vi "Scaled XOR Eval.vi"(11 "Neural Network Out":T1) -> (3 "3D Plot lvclass Array out":refnum<class "3D Plot Datatype.lvclass">[](array[class]))   [LabVIEW 2011, in "Super Simple Neural Network.lvlib"]
uses:
  Super Simple Neural Network.lvlib
  <vilib>/Math Plots/3D Math Plots/3D Surface/3D Surface Datatype/3D Surface Datatype.lvclass
  <vilib>/Math Plots/3D Math Plots/3D Surface/3D Surface Datatype/Public/Plot Helper (Vector).vi
  <vilib>/Math Plots/3D Math Plots/3D Plot/3D Plot Datatype/3D Plot Datatype.lvclass
  Types/2D Array.ctl
  Types/Scaling Info.ctl
  Types/Neural Network.ctl
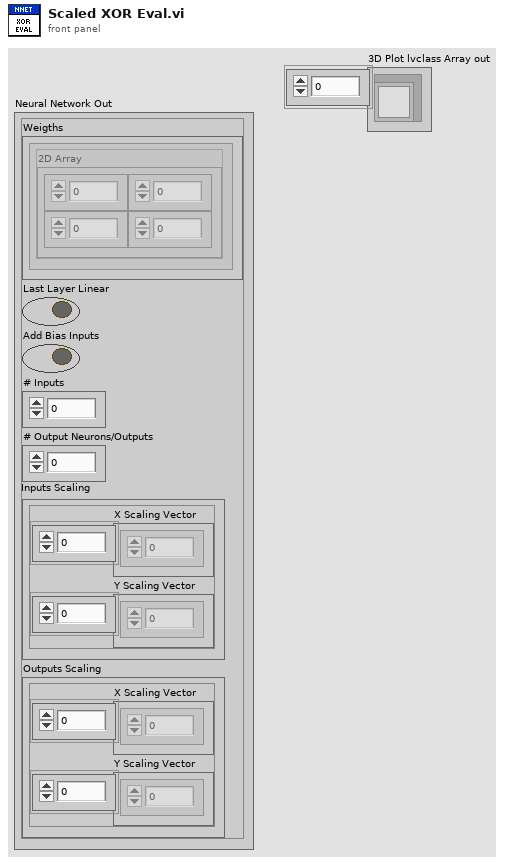
[diagram p1: front panel]
types:
  T1 = typedef "Super Simple Neural Network.lvlib/Neural Network.ctl" = cluster{"Weigths":T2[], "Last Layer Linear":bool, "Add Bias Inputs":bool, "# Inputs":u32, "# Output Neurons/Outputs":u32, "Inputs Scaling":T3, "Outputs Scaling":T3}
  T2 = typedef "Super Simple Neural Network.lvlib/2D Array.ctl" = cluster{"2D Array":dbl[][]}
  T3 = typedef "Super Simple Neural Network.lvlib/Scaling Info.ctl" = cluster{"X Scaling Vector":dbl[], "Y Scaling Vector":dbl[]}
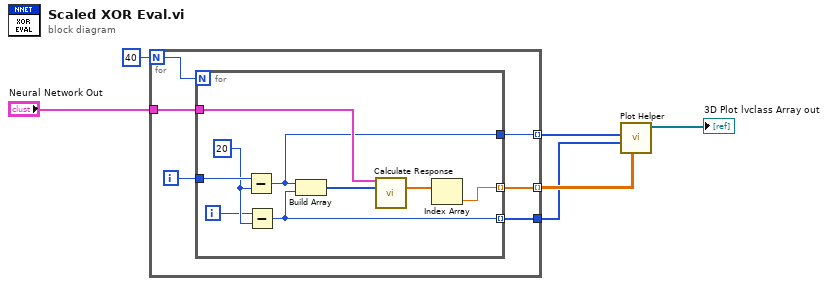
[diagram p0: block diagram]
diagram:
  n1 = for {
    N: 40 -> [w12]
    tunnel: "Neural Network Out" -> [w10]
    tunnel: [w9] -> w4 mode=indexing
    tunnel: [w8] -> w5
    tunnel: [w7] -> w6 mode=indexing
    i -> [w11]
    n2 = for {
      N: w12 -> [_]
      tunnel: w11 -> [w21]
      tunnel: w10 -> [w17]
      tunnel: [w16] -> w9
      tunnel: [w15] -> w8 mode=indexing
      tunnel: [w13] -> w7 mode=indexing
      i -> [w19]
      w20 = 20 ("y")
      n3 = Subtract(x=w21, y=w20) -> (x-y=w16:i32)
      n4 = Subtract(x=w19, y=w20) -> (x-y=w15:i32)
      n5 = Build Array(w16, w15) -> (w18:i32[])
      n6 = call "Calculate Response.vi"("Neural Network In"=w17, "Inputs"=w18) -> ("Outputs"=w14:dbl[])  [unwired: 11 in, 2 out]
      n7 = Index Array(array=w14) -> (element=w13:dbl)  [unwired: 1 in]
    }
  }
  n8 = call-poly <vilib>:"Plot Helper.vi"("z matrix"=w6, "y vector"=w5, "x vector"=w4) -> ("3D Plot lvclass Array out"=→"3D Plot lvclass Array out":refnum<class "3D Plot Datatype.lvclass">[])  [unwired: 3 in, 5 out]
